vi "GetStandardEventStatusEnableRegister.vi"(8 "Error In":errorcluster, 11 "Kiethley 2602 In":refnum<visa-resource-name>) -> (0 "Error Out":errorcluster, 2 "Standard Event Status Enable Register":bool[](array[boolean]), 3 "Keithley 2602 Out":refnum<visa-resource-name>)   [LabVIEW 2012, in "Keithley-2602.lvlib"]
uses:
  Keithley-2602.lvlib
panel:
  # "OPC"
  # "DDE"
  # "CME"
  # "PON"
  # "EXE"
  # "QYE"
  # "URQ"
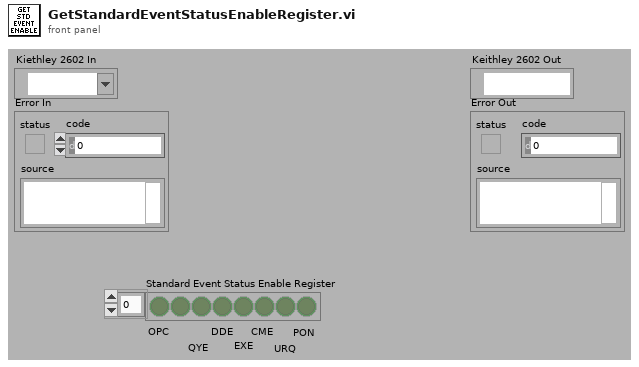
[diagram p1: front panel]
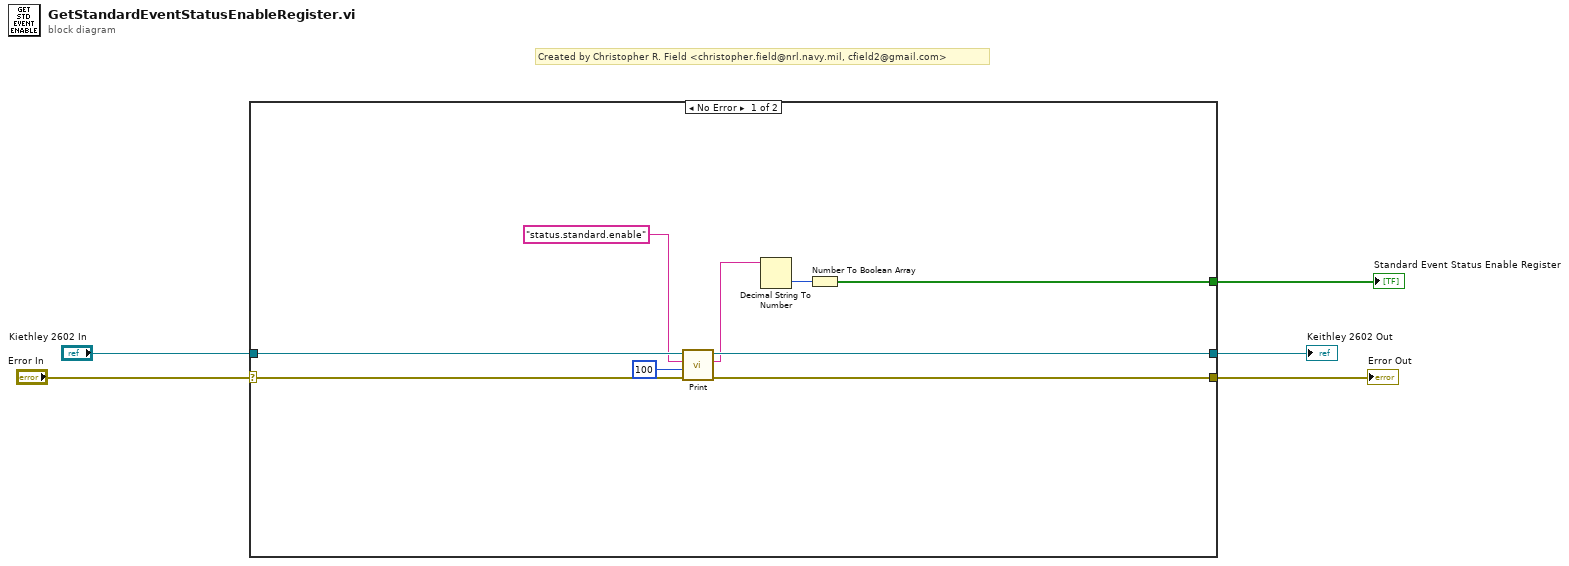
[diagram p0: block diagram]
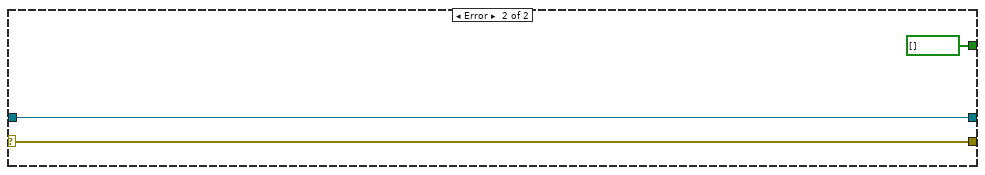
[diagram p2: hidden frame]
diagram:
  # "Created by Christopher R. Field <christopher.field@nrl.navy.mil, cfield2@gmail.com>"
  n1 = case shown="No Error" "Error In" {
    selector: "Error In" -> [w6 w16]
    tunnel: "Kiethley 2602 In" -> [w14 w17]
    tunnel: [w11 w17] -> w4
    tunnel: [w10 w16] -> w3
    tunnel: [w7 bool[] [] ("Boolean array")] -> w2
    frame No Error {
      n2 = call "Print.vi"("Error In"=w6, "Byte Count"=u32 100, "Attribute"="status.standard.enable", "Kiethley 2602 In"=w14) -> ("Error Out"=w10:errorcluster, "Output"=w9:string, "Keithley 2602 Out"=w11:refnum<visa-resource-name>)  [unwired: 5 in]
      n3 = Decimal String To Number(string=w9) -> (number=w8:i32)  [unwired: 2 in, 1 out]
      n4 = Number To Boolean Array(number=w8) -> (Boolean array=w7:bool[])
    }
    frame Error {
    }
  }
  "Keithley 2602 Out" <- w4
  "Error Out" <- w3
  "Standard Event Status Enable Register" <- w2
